vi "save and close project.vi"(8 "error in (no error)":errorcluster, 11 "Builders.lvclass":refnum<class "Builder.lvclass">) -> (0 "error out":errorcluster)   [LabVIEW 2024, in "Builder.lvclass"]
doc: "saves and closes the project reference"
uses:
  Builder.lvclass
  Builder.lvclass/Builder.ctl
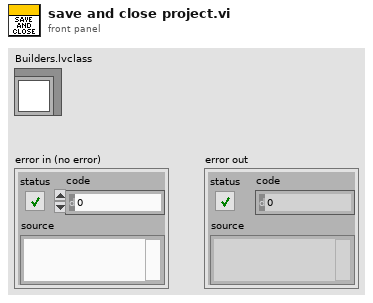
[diagram p1: front panel]
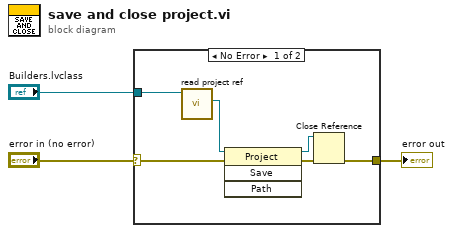
[diagram p0: block diagram]
diagram:
  n1 = case shown="No Error" "error in (no error)" {
    selector: "error in (no error)" -> [w9 w10]
    tunnel: [w6 w10] -> w2
    tunnel: "Builders.lvclass" -> [w5 _]
    frame No Error {
      n2 = call "read project ref.vi"("Builders in"=w5) -> ("project ref"=w4:refnum<vi>)  [unwired: 10 in]
      n3 = invoke class="Project" method="Save"(reference=w4, error in=w9) -> (reference out=w8:refnum<vi>, error out=w7:errorcluster)  [unwired: 2 in, 2 out]
      n4 = Close Reference(reference=w8, error in (no error)=w7) -> (error out=w6:errorcluster)
    }
    frame Error {
      # "#TODO\ndelete temp folder if build fails"
    }
  }
  "error out" <- w2
